vi "toString.vi"(8 "error in (no error)":errorcluster, 11 "BaseMessage in":refnum<class "BaseMessage.lvclass">) -> (0 "error out":errorcluster, 2 "String":string, 3 "BaseMessage out":refnum<class "BaseMessage.lvclass">)   [LabVIEW 2025, in "BaseMessage.lvclass"]
doc: "Format the message to a string. For each protocol that needs to be implemented. creata a child class of BaseMessage and overload this method"
uses:
  BaseMessage.lvclass
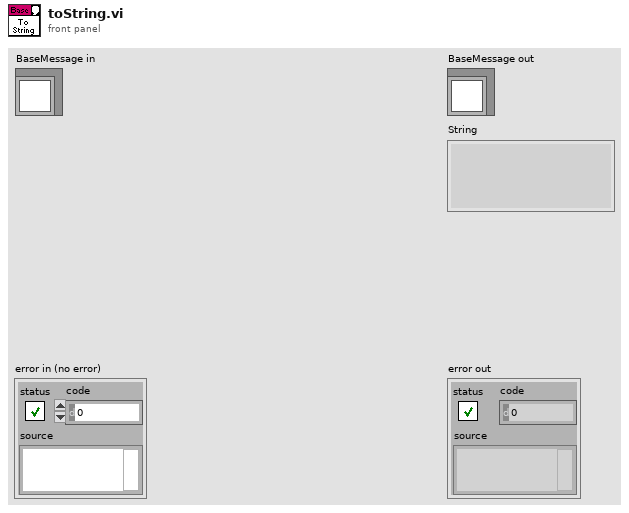
[diagram p1: front panel]
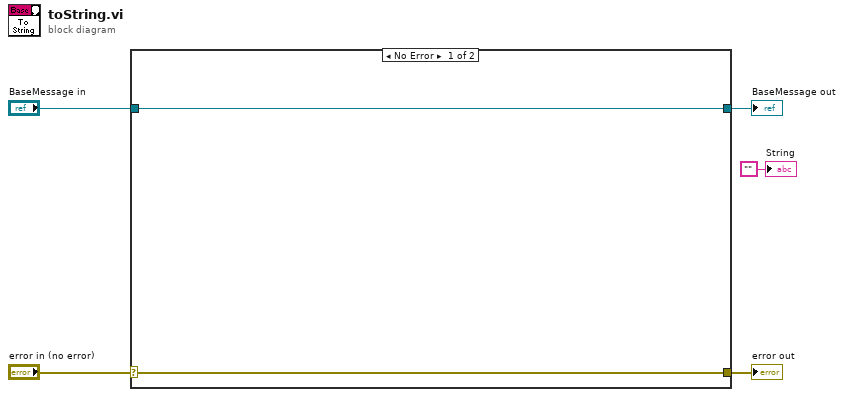
[diagram p0: block diagram]
diagram:
  n1 = case shown="No Error" "error in (no error)" {
    selector: "error in (no error)" -> [w6 w9]
    tunnel: [w6 w9] -> w4
    tunnel: [w7 w8] -> w2
    tunnel: "BaseMessage in" -> [w7 w8]
    frame No Error {
    }
    frame Error {
    }
  }
  "error out" <- w4
  "BaseMessage out" <- w2
  "String" <- "" ("String")
